vi "PROYECTO LENIN 2.vi"() -> ()   [LabVIEW 2025]
uses:
  <vilib>/MakerHub/LINX/Public/Peripherals/Analog/Analog Read 1 Chan.vi
  <vilib>/MakerHub/LINX/Public/Peripherals/Analog/Analog Read N Chans.vi
  <vilib>/MakerHub/LINX/Private/Local IO/LinxAnalogRead.vi
  <vilib>/MakerHub/LINX/Public/Utilities/Check Channel.vi
  <vilib>/MakerHub/LINX/Public/Utilities/Open Serial.vi
  <vilib>/MakerHub/LINX/Private/Utilties/Generate Error.vi
  <vilib>/MakerHub/LINX/LMH-LINX.lvlib
panel:
  in  "COM":refnum<visa-resource-name>
  out "BPM":dbl
  in  "STOP":bool
  out "PULSO":bool
  out "ECG":dbl(graph)
  out "PULSOS":dbl
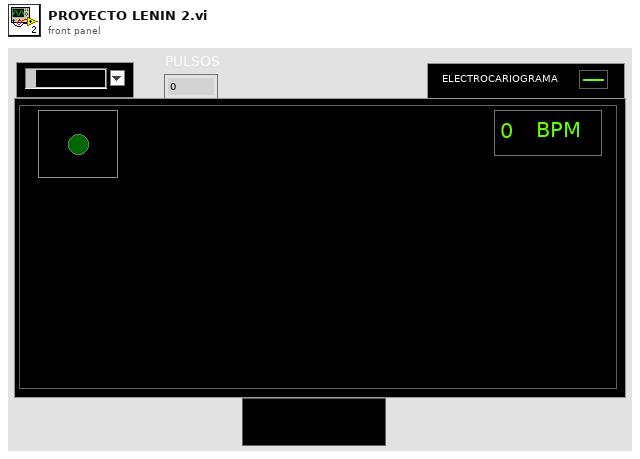
[diagram p1: front panel]
types:
  T1 = typedef "LMH-LINX.lvlib/LINX Ref.ctl" = cluster{"IO":T2, "Interface":T3, "LINX Device Config":T4}
  T2 = typedef "LMH-LINX.lvlib/Platform.ctl" = enum16{"Remote", "Local"}
  T3 = typedef "LMH-LINX.lvlib/Interface.ctl" = enum16{"Serial", "TCP"}
  T4 = typedef "LMH-LINX.lvlib/Device.lvlib/LINX Device Config.ctl" = cluster{"Interface":T3, "COM Port":refnum<visa-resource-name>, "TCP Configuration":T5, "Device Family":u8, "Device ID":u8, "Device Name":string, "TCP Ref":refnum<k5>, "Channels":T6}
  T5 = typedef "LMH-LINX.lvlib/Device.lvlib/TCP Config.ctl" = cluster{"IP Address":string, "Port":u16}
  T6 = typedef "LMH-LINX.lvlib/Channels.ctl" = cluster{"DI":u8[], "DO":u8[], "AI":u8[], "AO":u8[], "PWM":u8[], "QE":u8[], "UART":u8[], "I2C 2":u8[], "SPI":u8[], "CAN":u8[], "Servo":u8[], "AI Ref (V)":dbl, "AI Resolution (Bits)":u8, "AO Ref (V)":dbl, "AO Resolution (Bits)":u8}
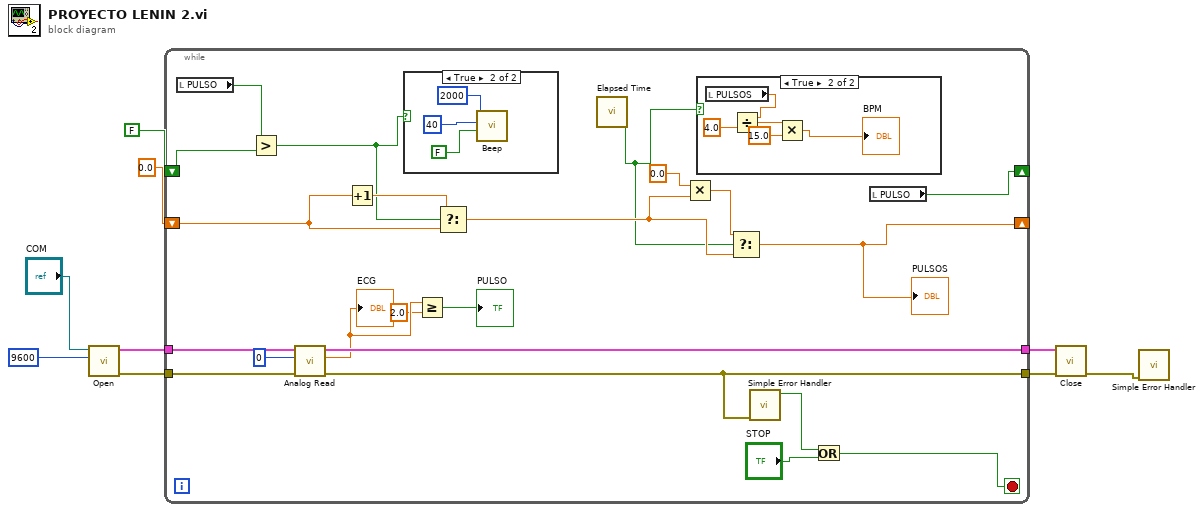
[diagram p0: block diagram]
diagram:
  n1 = call-poly <vilib>:"Open.vi"("Baud Rate Override"=u32 9600, "Serial Port"="COM") -> ("Error Out"=w8:errorcluster, "LINX Resource"=w9:T1)  [unwired: 7 in, 1 out]
  n2 = while {
    tunnel: w9 -> [w31]
    tunnel: w8 -> [w30]
    tunnel: [w21] -> w7
    tunnel: [w29] -> w6
    shift-right: [w11] -> _
    shift-left: FALSE -> [w15]
    shift-right: [w12] -> _
    shift-left: 0.0 -> [w16]
    stop <- w24 stop-if-true
    n3 = local read "PULSO"() -> (w14:bool)
    n4 = Greater?(x=w14, y=w15) -> (0:w10:bool)
    n5 = call-poly <vilib>:"Analog Read.vi"("Error In"=w30, "Analog Channel"=u8 0, "LINX Resource"=w31) -> ("Error Out"=w21:errorcluster, "Voltage"=w27:dbl, "LINX Resource"=w29:T1)  [unwired: 5 in, 1 out]
    "ECG" <- w27
    n6 = Increment(x=w16) -> (x+1=w17:dbl)
    n7 = case shown="True" w10 {
      frame False {
      }
      frame True {
        n8 = call <vilib>:"Beep.vi"("use system alert? (T)"=FALSE, "duration (msec)"=u32 40, "frequency (Hz)"=u32 2000) -> ()  [unwired: 9 in]
      }
    }
    n9 = Greater Or Equal?(x=w27, y=2.0) -> (x >= y?=→"PULSO":bool)
    n10 = Select(t=w17, s=w10, f=w16) -> (s? t:f=w19:dbl)
    n11 = call "Elapsed Time"() -> ("Time has Elapsed"=w13:bool)  [unwired: 12 in, 7 out]
    n12 = Multiply(x=0.0, y=w19) -> (x*y=w20:dbl)
    n13 = case shown="True" w13 {
      frame False {
      }
      frame True {
        n14 = local read "PULSOS"() -> (w39:dbl)
        n15 = Divide(x=w39, y=4.0) -> (x/y=w37:dbl)
        n16 = Multiply(x=w37, y=15.0) -> (x*y=→"BPM":dbl)
      }
    }
    n17 = Select(t=w20, s=w13, f=w19) -> (s? t:f=w12:dbl)
    "PULSOS" <- w12
    n18 = call <vilib>:"Simple Error Handler.vi"("error in (no error)"=w21) -> ("error?"=w22:bool)  [unwired: 4 in, 4 out]
    n19 = Or(x=w22, y="STOP") -> (x .or. y?=w24:bool)
    n20 = local read "PULSO"() -> (w11:bool)
  }
  n21 = call <vilib>:"Close.vi"("Error In"=w7, "LINX Resource"=w6) -> ("Error Out"=w3:errorcluster)  [unwired: 9 in]
  n22 = call <vilib>:"Simple Error Handler.vi"("error in (no error)"=w3) -> ()  [unwired: 4 in, 5 out]
